vi "setRowColor.vi"(8 "error in (no error)":errorcluster, 10 "Table in":refnum<vi>, 11 "reference in":refnum<class "Project Panels.lvclass">) -> (0 "error out":errorcluster, 3 "reference out":refnum<class "Project Panels.lvclass">)   [LabVIEW 2015, in "Project Panels.lvclass"]
uses:
  Project Panels.lvclass
  APP/excelFile_class/fileType.ctl
  SYS/File Controller_llb/File Controller.lvclass
  APP/excelFile_class/excelFile.lvclass
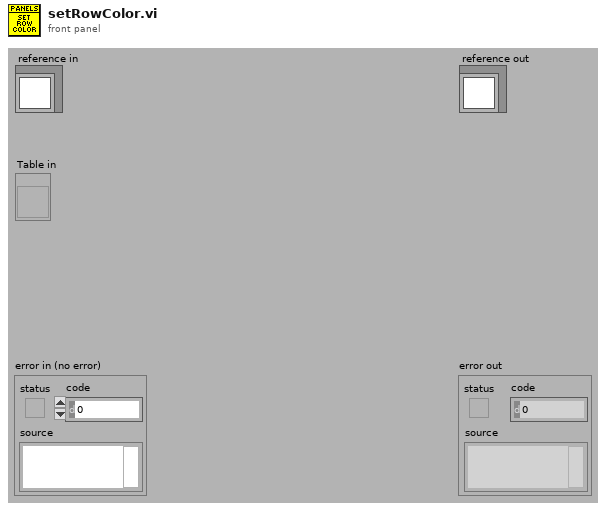
[diagram p1: front panel]
types:
  T1 = typedef "excelFile.lvclass/fileType.ctl" = enum16{"devices", "items", "partsTracking"}
  T2 = typedef "Project Panels.lvclass/ObjectAttributesRef.ctl" = refnum<data-value>
  T3 = typedef "Project Panels.lvclass/ObjectAttributes.ctl" = cluster{"MyAttribute":dbl, "device_controller_ref":refnum<class "Devices Controller.lvclass">, "file_controller_ref":refnum<class "File Controller.lvclass">, "item_controller_ref":refnum<class "Items Controller.lvclass">, "item_tables":cluster{"checkIN":string[][], "checkOUT":string[][], "storage":string[][]}, "quickbook_table":cluster{"notes":string[][]}, "notification_controller_ref":refnum<class "Notification Controller.lvclass">, "partstracking_controller_ref":refnum<class "PartsTracking Controller.lvclass">, "product_tables":cluster{"k4b2":string[][], "fitmate":string[][], "RMR":string[][], "CPET":string[][], "BP":string[][], "PP":string[][], "k5":string[][], "bb-pft":string[][]}, "rowsColour":u32[], "low_resolution?":bool}
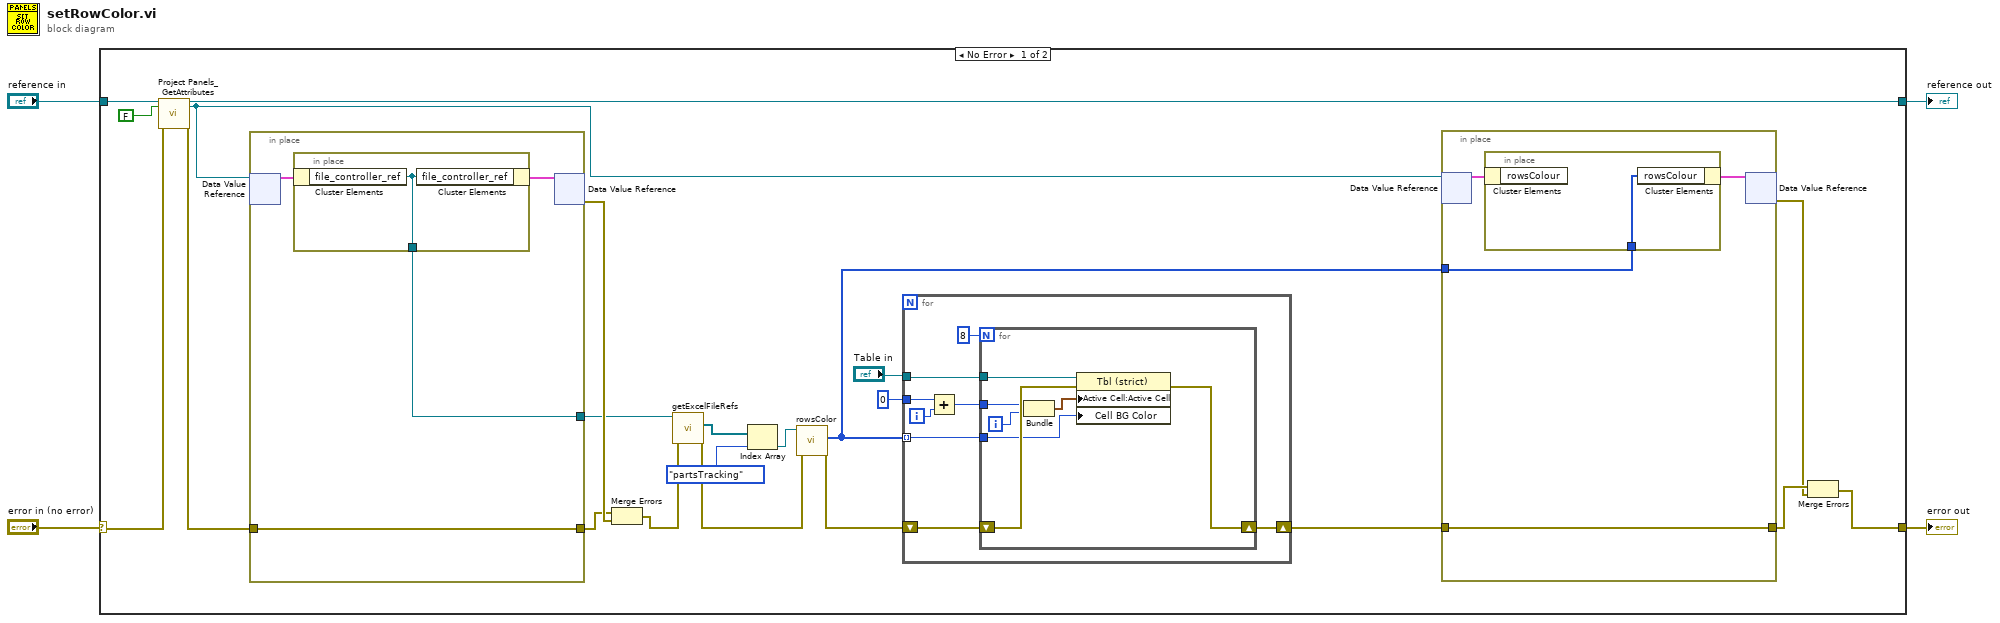
[diagram p0: block diagram]
diagram:
  n1 = case shown="No Error" "error in (no error)" {
    selector: "error in (no error)" -> [w22 w53]
    tunnel: [w7 w53] -> w3
    tunnel: [w20 w52] -> w1
    tunnel: "reference in" -> [w24 w52]
    frame No Error {
      n2 = call "Project Panels_GetAttributes.vi"("reference in"=w24, "return data? (T)"=FALSE, "error in (no error)"=w22) -> ("reference out"=w20:refnum<class "Project Panels.lvclass">, "attributes ref"=w6:T2, "error out"=w21:errorcluster)  [unwired: 13 in, 1 out]
      n3 = in-place {
        in-place-border: w21 -> [w48]
        in-place-border: [w48] -> w25
        in-place-border: [w47] -> w19
        n4 = in-place-dvr #1(w6) -> (w49:T3)  [unwired: 1 out]
        n5 = in-place {
          in-place-border: [w51] -> w47
          n6 = in-place-cluster #2(w49) -> ("file_controller_ref"=w51:refnum<class "File Controller.lvclass">)
          n7 = in-place-cluster #2("file_controller_ref"=w51) -> (w50:T3)
        }
        n8 = in-place-dvr #1(w50) -> (w26:errorcluster)  [unwired: 1 out]
      }
      n9 = Merge Errors(w25, w26) -> (w18:errorcluster)
      n10 = call "getExcelFileRefs.vi"("error in (no error)"=w18, "reference in"=w19) -> ("error out"=w14:errorcluster, "excelFile_refs"=w17:refnum<class "excelFile.lvclass">[])  [unwired: 7 in, 1 out]
      n11 = Index Array(array=w17, index=fileType."partsTracking" ("fileType")) -> (element=w15:refnum<class "excelFile.lvclass">)
      n12 = call "rowsColor.vi"("error in (no error)"=w14, "reference in"=w15) -> ("error out"=w12:errorcluster, "rowsColor"=w5:u32[])  [unwired: 7 in, 1 out]
      n13 = for {
        tunnel: "Table in" -> [w37]
        shift-right: [w38] -> w8
        shift-left: w12 -> [w39]
        tunnel: w5 -> [w35] mode=indexing
        tunnel: 0 -> [w34]
        i -> [w33]
        n14 = Add(x=w34, y=w33) -> (x+y=w32:i32)
        n15 = for {
          N: 8 -> [_]
          shift-right: [w45] -> w38
          shift-left: w39 -> [w46]
          tunnel: w32 -> [w43]
          tunnel: w37 -> [w44]
          tunnel: w35 -> [w40]
          i -> [w42]
          n16 = Bundle(w43, w42) -> (w41:cluster{i32, i32})  [unwired: 1 in]
          n17 = property on="Property Node" class="Tbl (strict)"(reference=w44, error in=w46, "Active Cell:Active Cell"=w41, "Cell BG Color"=w40) -> (error out=w45:errorcluster)  [unwired: 1 out]
        }
      }
      n18 = in-place {
        in-place-border: w8 -> [w28]
        in-place-border: [w28] -> w10
        in-place-border: w5 -> [w27]
        n19 = in-place-dvr #3(w6) -> (w29:T3)  [unwired: 1 out]
        n20 = in-place {
          in-place-border: w27 -> [w31]
          n21 = in-place-cluster #4(w29) -> ()  [unwired: 1 out]
          n22 = in-place-cluster #4("rowsColour"=w31) -> (w30:T3)
        }
        n23 = in-place-dvr #3(w30) -> (w9:errorcluster)  [unwired: 1 out]
      }
      n24 = Merge Errors(w10, w9) -> (w7:errorcluster)
    }
    frame Error {
    }
  }
  "error out" <- w3
  "reference out" <- w1
